vi "checkModbus.vi"(8 "error in (no error)":errorcluster, 11 "Mockbus in":refnum<class "Mockbus.lvclass">) -> (0 "error out":errorcluster, 3 "Mockbus out":refnum<class "Mockbus.lvclass">)   [LabVIEW 2015, in "Mockbus.lvclass"]
uses:
  Mockbus.lvclass
  Mockbus.lvclass/Mockbus.ctl
  Modbus/Modbus/Modbus.lvclass
  Utilities/FrameParser/FrameParser.lvclass
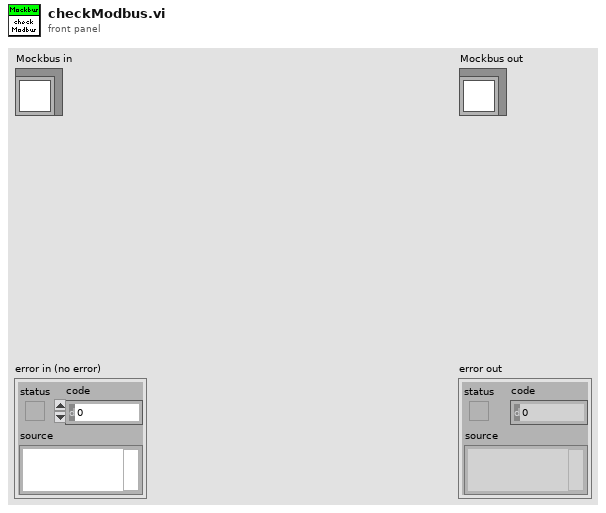
[diagram p1: front panel]
types:
  T1 = typedef "RTTypeDefs.lvlib/Frame.ctl" = cluster{"Data":u8[], "WaitForTrigger":bool, "WaitForRx":u16, "TriggerIRQ":i16}
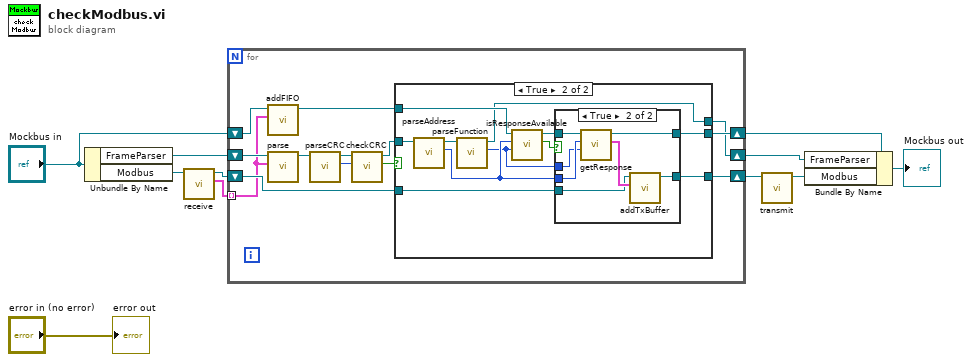
[diagram p0: block diagram]
diagram:
  n1 = Unbundle By Name("Mockbus in") -> ("FrameParser"=w2:refnum<class "FrameParser.lvclass">, "Modbus"=w11:refnum<class "Modbus.lvclass">)
  n2 = call "receive.vi"("Modbus in"=w11) -> ("Data"=w10:T1[], "Modbus out"=w8:refnum<class "Modbus.lvclass">)  [unwired: 8 in, 1 out]
  n3 = for {
    shift-right: [w20] -> w7
    shift-left: "Mockbus in" -> [w23]
    tunnel: w10 -> [w18] mode=indexing
    shift-right: [w21] -> w4
    shift-left: w8 -> [w22]
    shift-right: [w12] -> w1
    shift-left: w2 -> [w19]
    n4 = call "addFIFO.vi"("Frame"=w18, "Mockbus in"=w23) -> ("Mockbus out"=w24:refnum<class "Mockbus.lvclass">)  [unwired: 8 in, 1 out]
    n5 = call "parse.vi"("Frame"=w18, "FrameParser in"=w19) -> ("FrameParser out"=w14:refnum<class "FrameParser.lvclass">)  [unwired: 8 in, 1 out]
    n6 = call "parseCRC.vi"("FrameParser in"=w14) -> ("CRC"=w17:u16, "FrameParser out"=w15:refnum<class "FrameParser.lvclass">)  [unwired: 8 in, 1 out]
    n7 = call "checkCRC.vi"("CRC"=w17, "FrameParser in"=w15) -> ("Valid?"=w16:bool, "FrameParser out"=w13:refnum<class "FrameParser.lvclass">)  [unwired: 7 in, 1 out]
    n8 = case shown="True" w16 {
      tunnel: w24 -> [w26 w38]
      tunnel: w22 -> [w27 w35]
      tunnel: [w27 w34] -> w21
      tunnel: [w26 w33] -> w20
      tunnel: w13 -> [w25 w32]
      tunnel: [w25 w28] -> w12
      frame False {
      }
      frame True {
        n9 = call "parseAddress.vi"("FrameParser in"=w32) -> ("Address"=w30:u8, "FrameParser out"=w31:refnum<class "FrameParser.lvclass">)  [unwired: 8 in, 1 out]
        n10 = call "parseFunction.vi"("FrameParser in"=w31) -> ("Function"=w29:u8, "FrameParser out"=w28:refnum<class "FrameParser.lvclass">)  [unwired: 8 in, 1 out]
        n11 = call "isResponseAvailable.vi"("Function"=w29, "Address"=w30, "Mockbus in"=w38) -> ("Available?"=w37:bool, "Mockbus out"=w36:refnum<class "Mockbus.lvclass">)  [unwired: 6 in, 1 out]
        n12 = case shown="True" w37 {
          tunnel: w36 -> [w39 w46]
          tunnel: w35 -> [w40 w45]
          tunnel: [w40 w44] -> w34
          tunnel: [w39 w43] -> w33
          tunnel: w30 -> [_ w42]
          tunnel: w29 -> [_ w41]
          frame False {
          }
          frame True {
            n13 = call "getResponse.vi"("Function"=w41, "Address"=w42, "Mockbus in"=w46) -> ("Frame"=w47:T1, "Mockbus out"=w43:refnum<class "Mockbus.lvclass">)  [unwired: 6 in, 1 out]
            n14 = call "addTxBuffer.vi"("Frame"=w47, "Modbus in"=w45) -> ("Modbus out"=w44:refnum<class "Modbus.lvclass">)  [unwired: 8 in, 1 out]
          }
        }
      }
    }
  }
  n15 = call "transmit.vi"("Modbus in"=w4) -> ("Modbus out"=w3:refnum<class "Modbus.lvclass">)  [unwired: 9 in, 1 out]
  n16 = Bundle By Name(cluster=w7, "FrameParser"=w1, "Modbus"=w3) -> (→"Mockbus out":refnum<class "Mockbus.lvclass">)
  "error out" <- "error in (no error)"
